vi "Check First Instance Plugin.vi"(8 "error in (no error)":errorcluster, 11 "Plugin in":refnum<class "CSV Export.lvclass">) -> (0 "error out":errorcluster, 3 "Plugin out":refnum<class "CSV Export.lvclass">)   [LabVIEW 2022 SP3, in "CSV Export.lvlib" / "CSV Export.lvclass"]
uses:
  CSV Export.lvclass
  C:/Program Files/National Instruments/LabVIEW 2022/vi.lib/FlexLogger/SDK/PluginSDK.lvlibp/PEFClasses/SDK/Processing Element/Processing Element.lvclass
  <vilib>/FlexLogger/SDK/PluginSDK.lvlibp/PEFClasses/SDK/Processing Element/Read System Interface.vi
  <vilib>/FlexLogger/SDK/PluginSDK.lvlibp/PEFClasses/SDK/Processing Element/Read Alias.vi
  Global.vi
  <vilib>/FlexLogger/SDK/PluginSDK.lvlibp/PEFClasses/SDK/System Interface/System Interface.lvclass
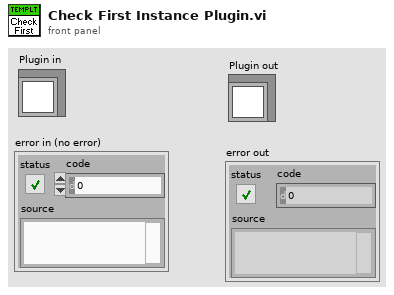
[diagram p1: front panel]
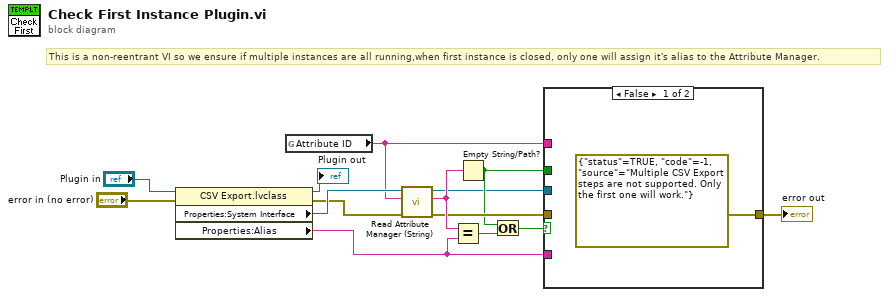
[diagram p0: block diagram]
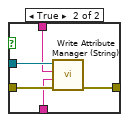
[diagram p3: hidden frame]
diagram:
  # "This is a non-reentrant VI so we ensure if multiple instances are all running,when first instance is closed, only one will assign it's alias to the Attribute Manager."
  n1 = property class="CSV Export.lvclass"(reference="Plugin in", error in="error in (no error)") -> (reference out=→"Plugin out":refnum<class "CSV Export.lvclass">, error out=w13:errorcluster, "Properties:System Interface"=w14:refnum<class "System Interface.lvclass">, "Properties:Alias"=w3:string)
  n2 = global read "Global.vi" "Attribute ID"() -> (w5:string)
  n3 = call-dynamic "Read Attribute Manager (String).vi"("error in (no error)"=w13, "Attribute ID"=w5, "System Interface in"=w14) -> ("error out"=w8:errorcluster, "Attrib Val"=w11:string, "System Interface out"=w4:refnum<class "System Interface.lvclass">)  [unwired: 5 in, 1 out]
  n4 = Equal?(x=w11, y=w3) -> (x = y?=w10:bool)
  n5 = Empty String/Path?(string/path=w11) -> (empty?=w6:bool)
  n6 = Or(x=w6, y=w10) -> (x .or. y?=w9:bool)
  n7 = case shown="False" w9 {
    tunnel: w8 -> [_ w20]
    tunnel: [errorcluster {"status"=TRUE, "code"=-1, "source"="Multiple CSV Export steps are not supported. Only the first one will work."} ("f") w16] -> w7
    tunnel: w6 -> [_ w17]
    tunnel: w5 -> [_ w19]
    tunnel: w4 -> [_ w21]
    tunnel: w3 -> [_ w18]
    frame False {
    }
    frame True {
      n8 = case shown="False" w17 {
        tunnel: w21 -> [_ w27]
        tunnel: w20 -> [w22 w26]
        tunnel: w19 -> [_ w25]
        tunnel: w18 -> [_ w24]
        tunnel: [w22 w23] -> w16
        frame False {
        }
        frame True {
          n9 = call-dynamic "Write Attribute Manager (String).vi"("error in (no error)"=w26, "Attribute Value"=w24, "Attribute ID"=w25, "System Interface in"=w27) -> ("error out"=w23:errorcluster)  [unwired: 5 in, 2 out]
        }
      }
    }
  }
  "error out" <- w7
